vi "Render Picture.vi"(11 "Graphic In":refnum<class "Graphic.lvclass">) -> (1 "Picture":picture, 3 "Graphic Out":refnum<class "Graphic.lvclass">)   [LabVIEW 2019, in "Graphic.lvclass"]
doc: "This VI is analogous to a pure virtual function. It does no real work and exists only to be overridden by its descendant classes."
uses:
  Graphic.lvclass
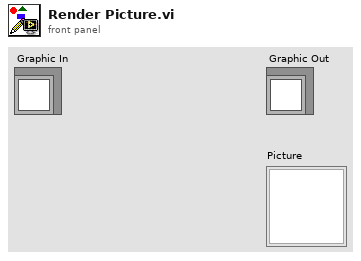
[diagram p1: front panel]
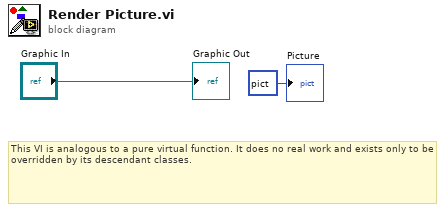
[diagram p0: block diagram]
diagram:
  # "This VI is analogous to a pure virtual function. It does no real work and exists only to be overridden by its descendant classes."
  "Picture" <- picture data[5B] ("Picture")
  "Graphic Out" <- "Graphic In"
